vi "XY Graph.vi"() -> ()   [LabVIEW 2023]
panel:
  out "error out 2":errorcluster
  in  "module path 2":path
  in  "Array 3":dbl[][](array[numeric])
  out "return value":dbl[][](array[numeric])
  out "XY Graph 3":cluster{"Y":dbl[], "Y":dbl[]}[](graph)
  out "XY Graph 2":cluster{"Y":dbl[], "Y":dbl[]}[](graph)
  out "XY Graph":cluster{"X":dbl[], "Y":dbl[]}[](graph)
  # "XY Graph"
  # "Lissajous Sin 3 hz  with Sin 4 Hz"
  # "Sin and cos with 90 start"
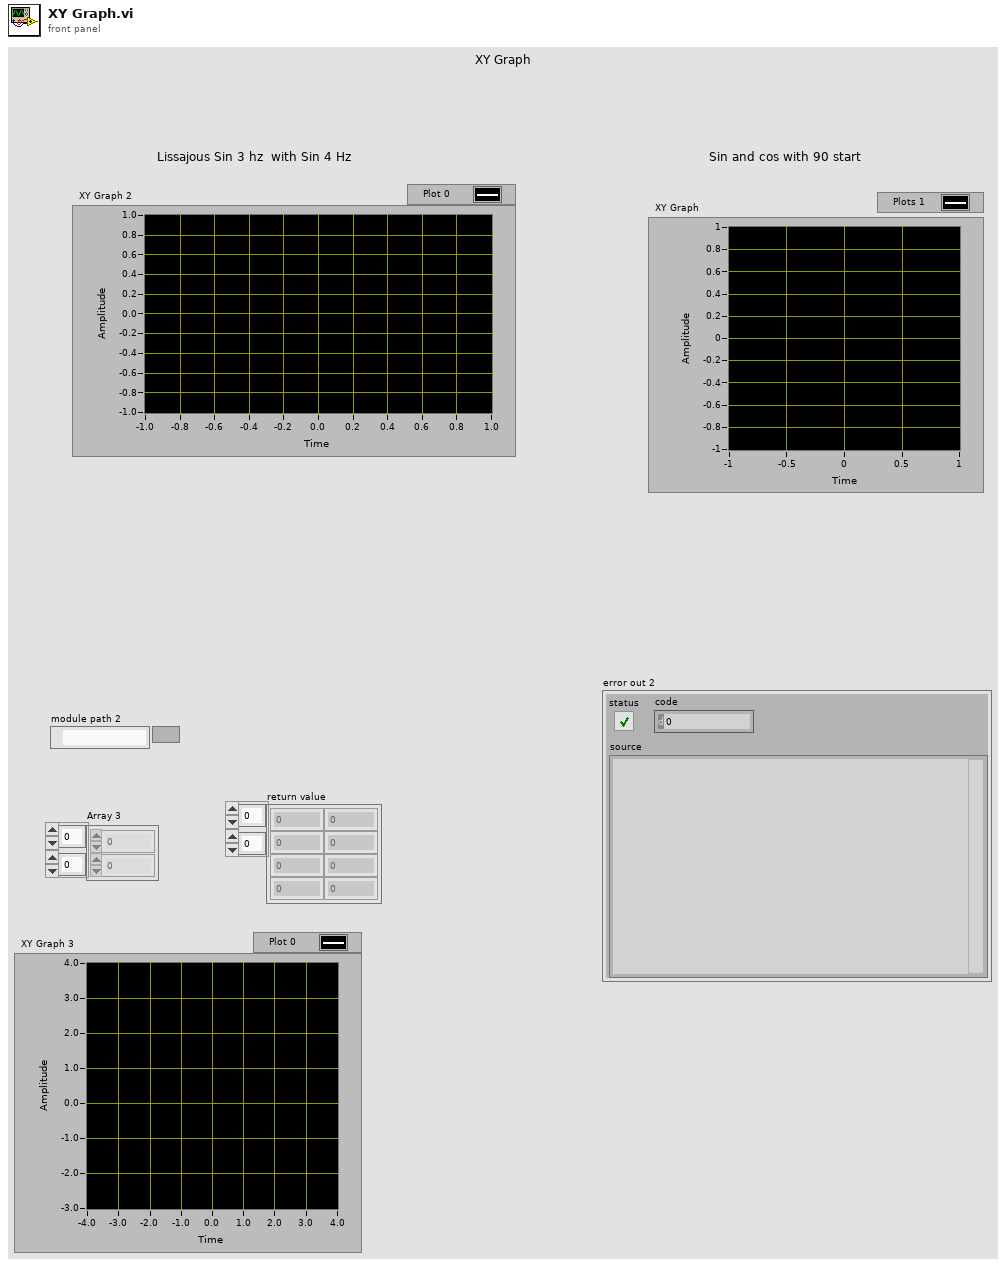
[diagram p1: front panel]
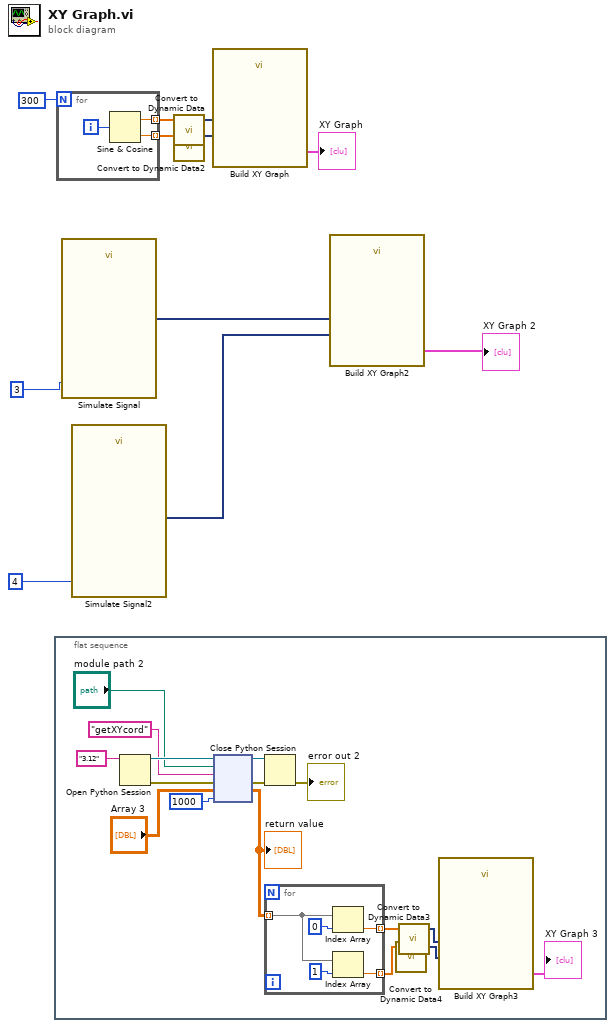
[diagram p0: block diagram]
diagram:
  n1 = flat-sequence {
    frame #0 {
      n2 = Open Python Session(python version="3.12" ("Python version")) -> (session out=w27:refnum<k35>, error out=w25:errorcluster)  [unwired: 2 in]
      n3 = node(w27, "module path 2", "getXYcord" ("function name"), w25, "Array 3", 1000) -> (w26:refnum<k35>, w24:errorcluster, w17:dbl[][])  [unwired: 1 in, 2 out]
      "return value" <- w17
      n4 = Close Python Session(session in=w26, error in=w24) -> (11:→"error out 2":errorcluster)
      n5 = for {
        tunnel: w17 -> [w31] mode=indexing
        tunnel: [w29] -> w15 mode=indexing
        tunnel: [w28] -> w13 mode=indexing
        n6 = Index Array(array=w31, index=0) -> (element=w29:dbl)
        n7 = Index Array(array=w31, index=1) -> (element=w28:dbl)
      }
      n8 = call "Convert to Dynamic Data4"("Array"=w13) -> ("Dynamic Data Type"=w12:dynamicdata)  [unwired: 3 in]
      n9 = call "Convert to Dynamic Data3"("Array"=w15) -> ("Dynamic Data Type"=w14:dynamicdata)  [unwired: 3 in]
      n10 = call "Build XY Graph3"("Y Input"=w12, "X Input"=w14) -> ("XY Graph"=→"XY Graph 3":cluster{"X":dbl[], "Y":dbl[]}[])  [unwired: 8 in, 1 out]
    }
  }
  n11 = for {
    N: 300 -> [_]
    tunnel: [w34] -> w10 mode=indexing
    tunnel: [w33] -> w8 mode=indexing
    i -> [w35]
    n12 = Sine & Cosine(0:w35) -> (1:w34:dbl, 2:w33:dbl)
  }
  n13 = call "Simulate Signal"("Frequency"=3) -> ("Sine"=w2:dynamicdata)  [unwired: 13 in, 1 out]
  n14 = call "Simulate Signal2"("Frequency"=4) -> ("Sine"=w1:dynamicdata)  [unwired: 13 in, 1 out]
  n15 = call "Convert to Dynamic Data"("Array"=w10) -> ("Dynamic Data Type"=w9:dynamicdata)  [unwired: 3 in]
  n16 = call "Convert to Dynamic Data2"("Array"=w8) -> ("Dynamic Data Type"=w7:dynamicdata)  [unwired: 3 in]
  n17 = call "Build XY Graph"("Y Input"=w7, "X Input"=w9) -> ("XY Graph"=→"XY Graph":cluster{"X":dbl[], "Y":dbl[]}[])  [unwired: 8 in, 1 out]
  n18 = call "Build XY Graph2"("Y Input"=w1, "X Input"=w2) -> ("XY Graph"=→"XY Graph 2":cluster{"X":dbl[], "Y":dbl[]}[])  [unwired: 8 in, 1 out]
